vi "Channel_Name_Options.vi"(0 "All Channel Names":string[](array[string]), 1 "Data string":string, 2 "Ignore When":string[][](array[string]), 5 "Template Names":string[](array[string]), 7 "Template File":path, 11 "Maths In":string[](array[string]), 12 "while Reading:":path, 13 "Filetype":string, 14 "Extra Channel Values":string[][](array[string])) -> (4 "Channels to find":string[](array[string]), 6 "Valid Channel Options":string[][](array[string]), 10 "Template updated?":bool)   [LabVIEW 2021]
uses:
  Controls/Global_mode.ctl
  Results_plotter_Global.vi
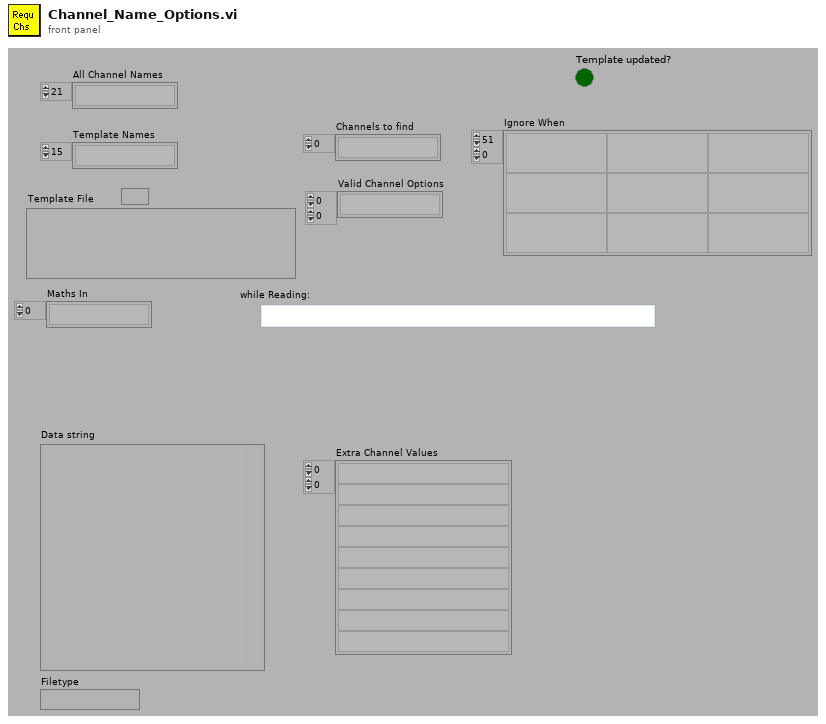
[diagram p1: front panel]
types:
  T1 = typedef "Global_mode.ctl" = enum16{"Read Global", "Load Global From File", "Write Global to File"}
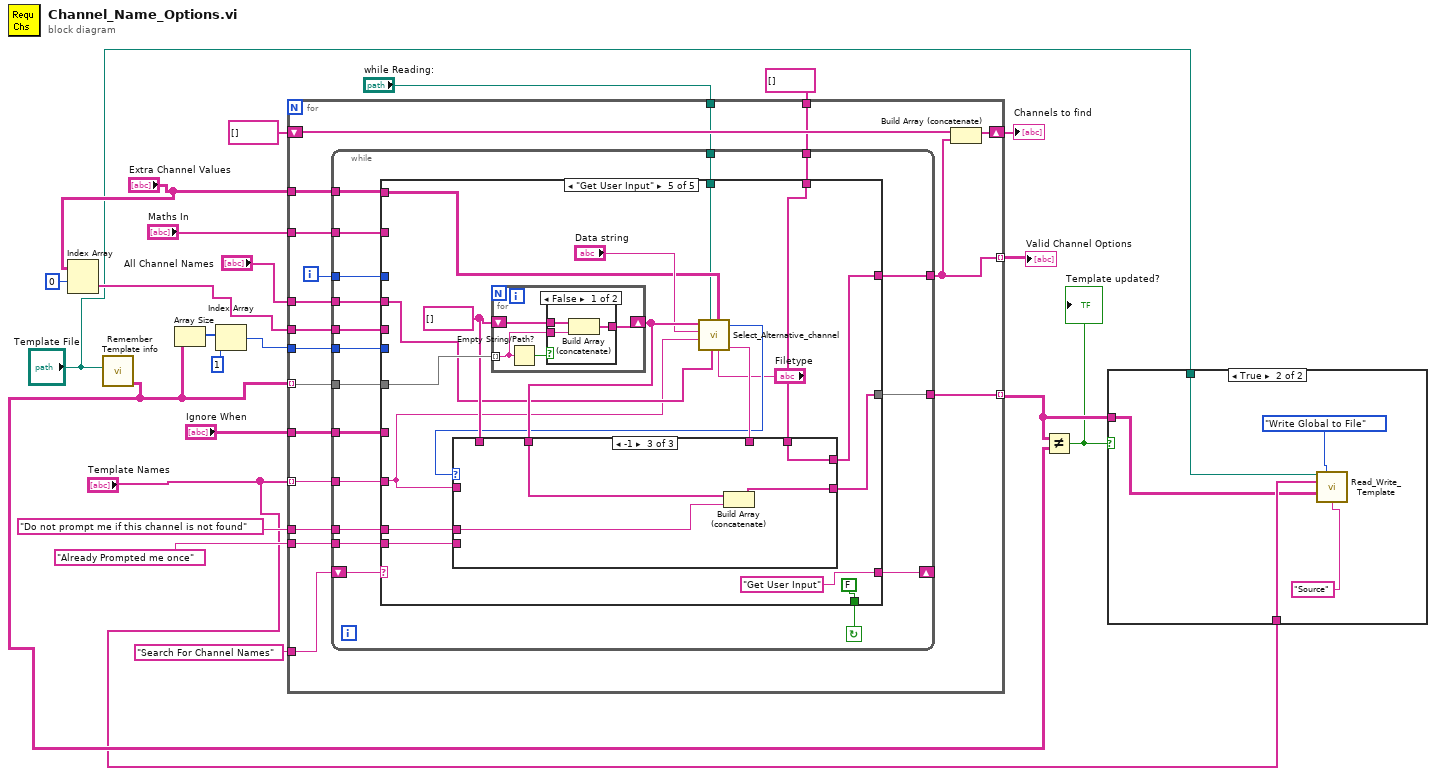
[diagram p0: block diagram]
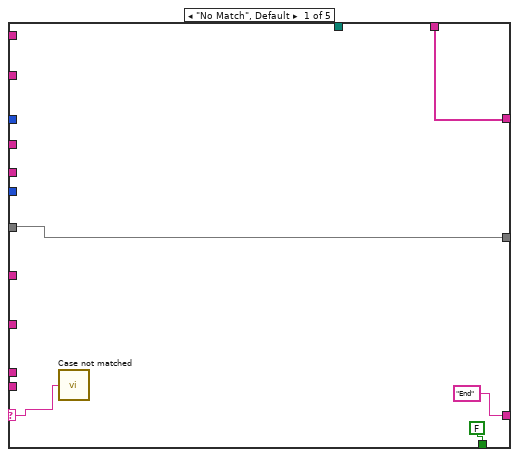
[diagram p3: hidden frame]
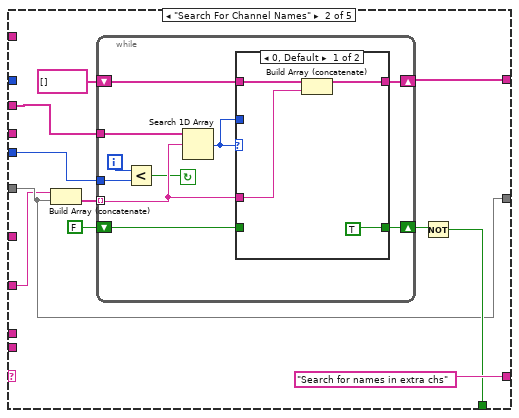
[diagram p4: hidden frame]
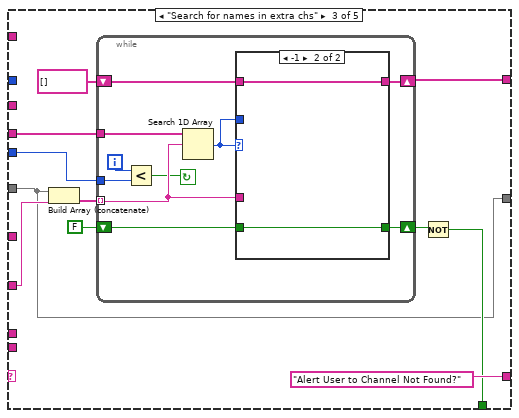
[diagram p6: hidden frame]
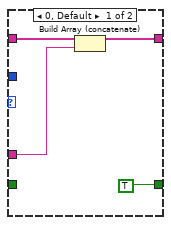
[diagram p7: hidden frame]
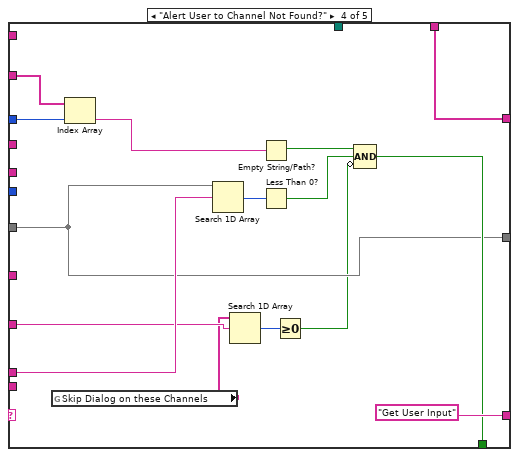
[diagram p8: hidden frame]
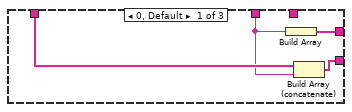
[diagram p9: hidden frame]
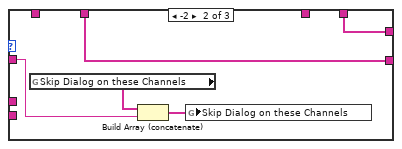
[diagram p10: hidden frame]
diagram:
  n1 = Index Array(array="Extra Channel Values", index (row)=0) -> (element=w7:string[])  [unwired: 1 in]
  n2 = call "Remember Template info.vi"("Template File"="Template File") -> ("Source"=w6:string[][])  [unwired: 6 in, 4 out]
  n3 = Array Size(array=w6) -> (size(s)=w22:i32[])
  n4 = Index Array(array=w22, index=1 ("Index")) -> (element=w20:i32)
  n5 = for {
    tunnel: "All Channel Names" -> [w40]
    tunnel: w6 -> [w38] mode=indexing
    tunnel: w20 -> [w39]
    tunnel: [w29] -> w17 mode=indexing
    tunnel: "Template Names" -> [w37] mode=indexing
    tunnel: [w36] -> w5 mode=indexing
    tunnel: "Do not prompt me if this channel is not found" -> [w35]
    tunnel: "Maths In" -> [w34]
    tunnel: "Search For Channel Names" -> [w32]
    shift-right: [w30] -> w15
    shift-left: string[] [] -> [w31]
    tunnel: string[] [] -> [w28]
    tunnel: w7 -> [w27]
    tunnel: "Already Prompted me once" -> [w26]
    tunnel: "Ignore When" -> [w25]
    tunnel: "Extra Channel Values" -> [w24]
    tunnel: "while Reading:" -> [w23]
    i -> [w33]
    n6 = while {
      tunnel: w27 -> [w45]
      tunnel: w28 -> [w46]
      tunnel: [w47] -> w29
      tunnel: w33 -> [w48]
      tunnel: w34 -> [w50]
      tunnel: w35 -> [w51]
      tunnel: [w52] -> w36
      tunnel: w37 -> [w53]
      tunnel: w38 -> [w56]
      tunnel: w39 -> [w57]
      tunnel: w40 -> [w58]
      shift-left: w32 -> [w49]
      shift-right: [w54] -> _
      tunnel: w26 -> [w44]
      tunnel: w25 -> [w43]
      tunnel: w24 -> [w42]
      tunnel: w23 -> [w41]
      stop <- w55 continue-if-true
      n7 = case shown="\"Get User Input\"" w49 {
        selector: w49 -> [w59 _ _ _ _]
        tunnel: w58 -> [_ w65 _ _ w140]
        tunnel: w57 -> [_ w74 w101 _ _]
        tunnel: w56 -> [w61 w66 w92 w122 w150]
        tunnel: [w60 w70 w97 w123 w147] -> w47
        tunnel: [FALSE w68 w95 w127 FALSE] -> w55
        tunnel: ["End" "Search for names in extra chs" "Alert User to Channel Not Found?" "Get User Input" "Get User Input"] -> w54
        tunnel: w53 -> [_ w64 w94 w119 w134]
        tunnel: [w61 w66 w92 w122 w148] -> w52
        tunnel: w51 -> [_ _ _ w131 w137]
        tunnel: w50 -> [_ _ _ w126 _]
        tunnel: w48 -> [_ _ _ w125 _]
        tunnel: w46 -> [w60 _ _ w123 w142]
        tunnel: w45 -> [_ _ w91 _ _]
        tunnel: w44 -> [_ _ _ _ w136]
        tunnel: w43 -> [_ _ _ _ _]
        tunnel: w42 -> [_ _ _ _ w135]
        tunnel: w41 -> [_ _ _ _ w133]
        frame "No Match", Default {
          n8 = call "Case not matched.vi"("Case Name not Matched"=w59) -> ()
        }
        frame "Search For Channel Names" {
          n9 = Build Array (concatenate)(w64, w66) -> (w67:string[])
          n10 = while {
            shift-left: string[] [] -> [w76]
            shift-right: [w79] -> w70
            shift-left: FALSE ("index of element") -> [w77]
            shift-right: [w78] -> w69
            tunnel: w67 -> [w81] mode=indexing
            tunnel: w74 -> [w82]
            tunnel: w65 -> [w84]
            i -> [w83]
            stop <- w75 continue-if-true
            n11 = Less?(x=w83, y=w82) -> (x < y?=w75:bool)
            n12 = Search 1D Array(1D array=w84, element=w81) -> (index of element=w80:i32)  [unwired: 1 out]
            n13 = case shown="0, Default" w80 {
              tunnel: w81 -> [w86 _]
              tunnel: w80 -> [_ _]
              tunnel: [w87 w89] -> w79
              tunnel: [TRUE w90] -> w78
              tunnel: w77 -> [_ w90]
              tunnel: w76 -> [w88 w89]
              frame 0, Default {
                n14 = Build Array (concatenate)(w88, w86) -> (w87:string[])
              }
              frame -1 {
              }
            }
          }
          n15 = Not(x=w69) -> (.not. x?=w68:bool)
        }
        frame "Search for names in extra chs" {
          n16 = Build Array (concatenate)(w92, w94) -> (w93:string[])
          n17 = while {
            shift-left: string[] [] -> [w103]
            shift-right: [w106] -> w97
            shift-left: FALSE ("index of element") -> [w104]
            shift-right: [w105] -> w96
            tunnel: w93 -> [w108] mode=indexing
            tunnel: w101 -> [w109]
            tunnel: w91 -> [w111]
            i -> [w110]
            stop <- w102 continue-if-true
            n18 = Less?(x=w110, y=w109) -> (x < y?=w102:bool)
            n19 = Search 1D Array(1D array=w111, element=w108) -> (index of element=w107:i32)  [unwired: 1 out]
            n20 = case shown="-1" w107 {
              tunnel: w108 -> [w113 _]
              tunnel: w107 -> [_ _]
              tunnel: [w114 w116] -> w106
              tunnel: [TRUE w117] -> w105
              tunnel: w104 -> [_ w117]
              tunnel: w103 -> [w115 w116]
              frame 0, Default {
                n21 = Build Array (concatenate)(w115, w113) -> (w114:string[])
              }
              frame -1 {
              }
            }
          }
          n22 = Not(x=w96) -> (.not. x?=w95:bool)
        }
        frame "Alert User to Channel Not Found?" {
          n23 = global read "Results_plotter_Global.vi" "Skip Dialog on these Channels"() -> (w118:string[])
          n24 = Index Array(array=w126, index=w125) -> (element=w124:string)
          n25 = Search 1D Array(1D array=w122, element=w131) -> (index of element=w132:i32)  [unwired: 1 out]
          n26 = Search 1D Array(1D array=w118, element=w119) -> (index of element=w121:i32)  [unwired: 1 out]
          n27 = Empty String/Path?(string/path=w124) -> (empty?=w129:bool)
          n28 = Less Than 0?(x=w132) -> (x < 0?=w128:bool)
          n29 = Greater Or Equal To 0?(x=w121) -> (x >= 0?=w120:bool)
          n30 = Compound Arithmetic op=AND(w129, w128, invert w120) -> (w127:bool)
        }
        frame "Get User Input" {
          w144 = string[] []
          n31 = for {
            shift-right: [w164] -> w146
            shift-left: w144 -> [w166]
            tunnel: w150 -> [w165] mode=indexing
            n32 = Empty String/Path?(string/path=w165) -> (empty?=w167:bool)
            n33 = case shown="False" w167 {
              tunnel: w166 -> [w170 w171]
              tunnel: [w169 w171] -> w164
              tunnel: w165 -> [w168 _]
              frame False {
                n34 = Build Array (concatenate)(w170, w168) -> (w169:string[])
              }
              frame True {
              }
            }
          }
          n35 = call "Select_Alternative_channel.vi"("Filetype"="Filetype", "Extra Channel Values"=w135, "All Tabulated Channels"=w140, "while Reading:"=w133, "Template Channel Name"=w134, "Data string"="Data string", "Previous Channels used"=w146) -> ("Chosen Channel"=w145:string, "Selected Index"=w141:i32)  [unwired: 3 in]
          n36 = case shown="-1" w141 {
            tunnel: [w154 w158 w163] -> w148
            tunnel: [w151 w159 w162] -> w147
            tunnel: w146 -> [w153 w158 w161]
            tunnel: w145 -> [w152 _ _]
            tunnel: w144 -> [_ _ _]
            tunnel: w142 -> [_ w159 w162]
            tunnel: w137 -> [_ _ w160]
            tunnel: w136 -> [_ _ _]
            tunnel: w134 -> [_ w156 _]
            frame 0, Default {
              n37 = Build Array(w152) -> (w151:string[])
              n38 = Build Array (concatenate)(w153, w152) -> (w154:string[])
            }
            frame -2 {
              n39 = global read "Results_plotter_Global.vi" "Skip Dialog on these Channels"() -> (w157:string[])
              n40 = Build Array (concatenate)(w157, w156) -> (w155:string[])
              n41 = global write "Results_plotter_Global.vi" "Skip Dialog on these Channels"(w155) -> ()
            }
            frame -1 {
              n42 = Build Array (concatenate)(w161, w160) -> (w163:string[])
            }
          }
        }
      }
    }
    n43 = Build Array (concatenate)(w31, w29) -> (w30:string[])
  }
  "Valid Channel Options" <- w17
  "Channels to find" <- w15
  n44 = Not Equal?(x=w5, y=w6) -> (x != y?=w4:bool)
  "Template updated?" <- w4
  n45 = case shown="True" w4 {
    tunnel: w5 -> [_ w172]
    tunnel: "Template Names" -> [_ w176]
    tunnel: "Template File" -> [_ w175]
    frame False {
    }
    frame True {
      n46 = call "Read_Write_Template.vi"("Template File"=w175, "Mode"=Global_mode."Write Global to File", "Channel names In"=w176, "2D Info In"=w172, "Data type"="Source") -> ()  [unwired: 3 in, 8 out]
    }
  }
